vi "Get Space Coordinates.vi"(8 "Visualizer Zoom":cluster{"X":i32, "Y":i32}, 9 "coordinates [pix]":cluster{"X":sgl, "Y":sgl} {"Y" format="%.2f"; "X" format="%.2f"}, 10 "FOV":cluster{"X [um]":dbl, "Y [um]":dbl} {"Y [um]" format="%.2f"; "X [um]" format="%.2f"}, 11 "Image Area":cluster{"Width":u32, "Height":u32}) -> (2 "coordinates [pix]":cluster{"X":sgl, "Y":sgl} {"Y" format="%.2f"; "X" format="%.2f"}, 3 "coordinates [um]":cluster{"X [um]":dbl, "Y [um]":dbl})   [LabVIEW 2012, in "Targeting Unit.lvlib"]
uses:
  Targeting Unit.lvlib
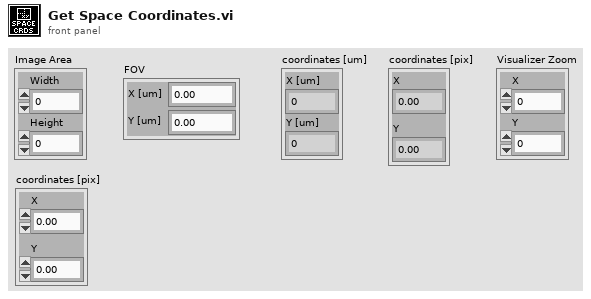
[diagram p1: front panel]
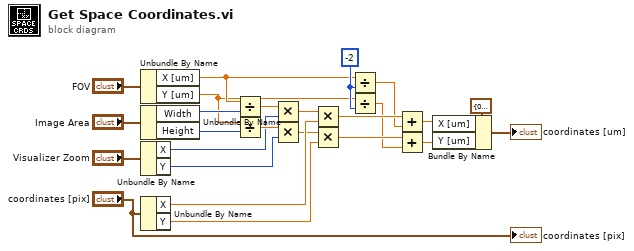
[diagram p0: block diagram]
diagram:
  w9 = -2 ("y")
  n1 = Unbundle By Name("FOV") -> ("X [um]"=w2:dbl, "Y [um]"=w1:dbl)
  n2 = Unbundle By Name("Image Area") -> ("Width"=w21:u32, "Height"=w20:u32)
  n3 = Unbundle By Name("Visualizer Zoom") -> ("X"=w11:i32, "Y"=w10:i32)
  n4 = Unbundle By Name("coordinates [pix]") -> ("X"=w25:sgl, "Y"=w19:sgl)
  n5 = Divide(x=w2, y=w21) -> (x/y=w16:dbl)
  n6 = Divide(x=w1, y=w20) -> (x/y=w15:dbl)
  n7 = Multiply(x=w16, y=w11) -> (x*y=w14:dbl)
  n8 = Multiply(x=w15, y=w10) -> (x*y=w13:dbl)
  n9 = Multiply(x=w14, y=w25) -> (x*y=w8:dbl)
  n10 = Multiply(x=w13, y=w19) -> (x*y=w7:dbl)
  n11 = Divide(x=w2, y=w9) -> (x/y=w4:dbl)
  n12 = Divide(x=w1, y=w9) -> (x/y=w3:dbl)
  n13 = Add(x=w8, y=w4) -> (x+y=w6:dbl)
  n14 = Add(x=w7, y=w3) -> (x+y=w5:dbl)
  n15 = Bundle By Name(cluster=cluster{"X [um]":dbl, "Y [um]":dbl} {"X [um]"=0.0, "Y [um]"=0.0} ("input cluster"), "X [um]"=w6, "Y [um]"=w5) -> (→"coordinates [um]":cluster{"X [um]":dbl, "Y [um]":dbl})
  "coordinates [pix]" <- "coordinates [pix]"
